vi "ProcessDataV1729A_withPedSub.vi"(9 "Buffer":u32[](array[numeric]), 10 "TRIG_REC":u32, 11 "# Samples after Trig":u16) -> (0 "Channel Data":u16[][](array[numeric]), 1 "PedSubChnData":dbl[][](array[numeric]), 3 "Vernier Data":u16[](array[numeric]))   [LabVIEW 2014]
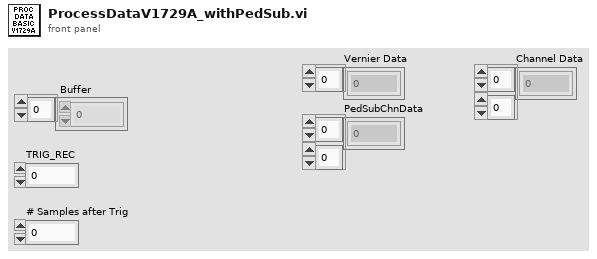
[diagram p1: front panel]
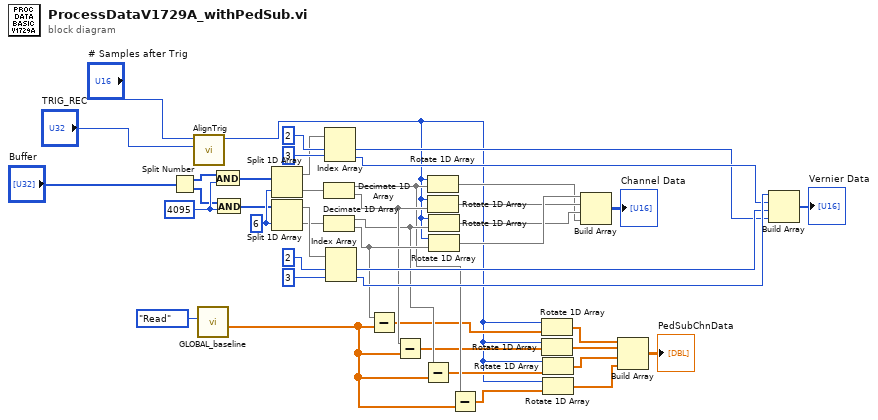
[diagram p0: block diagram]
diagram:
  w35 = 6 ("index")
  w32 = u16 4095 ("Numeric")
  n1 = Split Number(x="Buffer") -> (hi(x)=w31:u16[], lo(x)=w30:u16[])
  n2 = call "AlignTrig.vi"("TRIG_REC"="TRIG_REC", "# Samples after Trig"="# Samples after Trig") -> ("Offset"=w6:u16)  [unwired: 9 in]
  n3 = call "GLOBAL_baseline.vi"("State"=enum16{"Initialise", "Write", "Read"}."Read") -> ("Data out"=w11:dbl[])  [unwired: 10 in]
  n4 = And(x=w31, y=w32) -> (x .and. y?=w33:u16[])
  n5 = And(x=w30, y=w32) -> (x .and. y?=w34:u16[])
  n6 = Split 1D Array(array=w33, index=w35) -> (first subarray=w38:u16[], second subarray=w36:u16[])
  n7 = Split 1D Array(array=w34, index=w35) -> (first subarray=w41:u16[], second subarray=w37:u16[])
  n8 = Decimate 1D Array(w36) -> (w12:u16[], w14:u16[])
  n9 = Decimate 1D Array(w37) -> (w13:u16[], w15:u16[])
  n10 = Index Array(array=w38, index #1=2 ("index"), index #2=3 ("index")) -> (element #1=w18:u16, element #2=w20:u16)
  n11 = Index Array(array=w41, index #1=2 ("index"), index #2=3 ("index")) -> (element #1=w19:u16, element #2=w21:u16)
  n12 = Subtract(x=w15, y=w11) -> (x-y=w10:dbl[])
  n13 = Subtract(x=w14, y=w11) -> (x-y=w9:dbl[])
  n14 = Subtract(x=w13, y=w11) -> (x-y=w8:dbl[])
  n15 = Rotate 1D Array(1:w12, 2:w6) -> (0:w23:u16[])
  n16 = Rotate 1D Array(1:w14, 2:w6) -> (0:w25:u16[])
  n17 = Rotate 1D Array(1:w13, 2:w6) -> (0:w24:u16[])
  n18 = Rotate 1D Array(1:w15, 2:w6) -> (0:w26:u16[])
  n19 = Subtract(x=w12, y=w11) -> (x-y=w7:dbl[])
  n20 = Rotate 1D Array(1:w10, 2:w6) -> (0:w5:dbl[])
  n21 = Rotate 1D Array(1:w9, 2:w6) -> (0:w4:dbl[])
  n22 = Rotate 1D Array(1:w8, 2:w6) -> (0:w3:dbl[])
  n23 = Rotate 1D Array(1:w7, 2:w6) -> (0:w2:dbl[])
  n24 = Build Array(w26, w25, w24, w23) -> (→"Channel Data":u16[][])
  n25 = Build Array(w5, w4, w3, w2) -> (→"PedSubChnData":dbl[][])
  n26 = Build Array(w21, w20, w19, w18) -> (→"Vernier Data":u16[])
